vi "大富翁.vi"() -> ()   [LabVIEW 2014] (continued)
                        n3735 = local write "29旅1"(TRUE) -> ()
                      }
                      frame #1 {
                        n3736 = property on="29旅1" class="Bool (strict)"("Visible"=TRUE) -> ()  [unwired: 2 in, 2 out]
                      }
                    }
                  }
                  frame 6 {
                    n3737 = flat-sequence {
                      frame #0 {
                        n3738 = local write "29旅2"(TRUE) -> ()
                      }
                      frame #1 {
                        n3739 = property on="29旅2" class="Bool (strict)"("Visible"=TRUE) -> ()  [unwired: 2 in, 2 out]
                      }
                    }
                  }
                  frame 7 {
                    n3740 = flat-sequence {
                      frame #0 {
                        n3741 = local write "29旅3"(TRUE) -> ()
                      }
                      frame #1 {
                        n3742 = property on="29旅3" class="Bool (strict)"("Visible"=TRUE) -> ()  [unwired: 2 in, 2 out]
                      }
                    }
                  }
                  frame 8 {
                    n3743 = flat-sequence {
                      frame #0 {
                        n3744 = local write "29旅4"(TRUE) -> ()
                      }
                      frame #1 {
                        n3745 = property on="29旅4" class="Bool (strict)"("Visible"=TRUE) -> ()  [unwired: 2 in, 2 out]
                      }
                    }
                  }
                }
                n3746 = case shown="1, Default" w3039 {
                  tunnel: w3043 -> [w3075 w3076 w3077 w3078]
                  frame 1, Default {
                    n3747 = local write "玩家一財產"(w3075) -> ()
                  }
                  frame 2 {
                    n3748 = local write "玩家二財產"(w3076) -> ()
                  }
                  frame 3 {
                    n3749 = local write "玩家三財產"(w3077) -> ()
                  }
                  frame 4 {
                    n3750 = local write "玩家四財產"(w3078) -> ()
                  }
                }
              }
              frame True {
                # "無主地"
                n3751 = call "購買土地.vi"() -> ("確定 2"=w3085:bool)  [unwired: 3 in]
                n3752 = case shown="True" w3085 {
                  tunnel: w3084 -> [_ w3089]
                  frame False {
                    # "不買"
                  }
                  frame True {
                    # "要買"
                    n3753 = local read "換誰?"() -> (w3090:dbl)
                    n3754 = case shown="4" w3090 {
                      tunnel: [w3117 w3118 w3119 w3120] -> w3088
                      frame 1, Default {
                        n3755 = local read "玩家一財產"() -> (w3117:dbl)
                      }
                      frame 2 {
                        n3756 = local read "玩家二財產"() -> (w3118:dbl)
                      }
                      frame 3 {
                        n3757 = local read "玩家三財產"() -> (w3119:dbl)
                      }
                      frame 4 {
                        n3758 = local read "玩家四財產"() -> (w3120:dbl)
                      }
                    }
                    n3759 = call "各種價格.vi"("Numeric"=w3089) -> ("買空地"=w3087:dbl)  [unwired: 4 in, 5 out]
                    n3760 = Greater Or Equal?(x=w3088, y=w3087) -> (x >= y?=w3086:bool)
                    n3761 = case shown="True" w3086 {
                      tunnel: w3089 -> [_ w3091]
                      frame False {
                        # "錢不夠"
                        n3762 = call "錢不夠.vi"() -> ()  [unwired: 4 in]
                      }
                      frame True {
                        # "錢夠"
                        n3763 = local read "換誰?"() -> (w3092:dbl)
                        n3764 = case shown="3" w3092 {
                          selector: w3092 -> [w3096 w3102 w3108 w3114]
                          tunnel: w3091 -> [w3095 w3101 w3107 w3113]
                          frame 1, Default {
                            # "誰買了地"
                            n3765 = call "各種價格.vi"("Numeric"=w3095) -> ("買空地"=w3094:dbl)  [unwired: 4 in, 5 out]
                            n3766 = local read "玩家一財產"() -> (w3098:dbl)
                            n3767 = Subtract(x=w3098, y=w3094) -> (x-y=w3097:dbl)
                            n3768 = local write "玩家一財產"(w3097) -> ()
                            n3769 = call "數字轉顏色.vi"("數字"=w3096) -> ("顏色數字"=w3093:dbl)  [unwired: 2 in]
                            n3770 = local write "29彰化縣"(w3093) -> ()
                            n3771 = local write "彰化縣所有"(w3093) -> ()
                          }
                          frame 2 {
                            # "誰買了地"
                            n3772 = call "各種價格.vi"("Numeric"=w3101) -> ("買空地"=w3100:dbl)  [unwired: 4 in, 5 out]
                            n3773 = local read "玩家二財產"() -> (w3104:dbl)
                            n3774 = Subtract(x=w3104, y=w3100) -> (x-y=w3103:dbl)
                            n3775 = local write "玩家二財產"(w3103) -> ()
                            n3776 = call "數字轉顏色.vi"("數字"=w3102) -> ("顏色數字"=w3099:dbl)  [unwired: 2 in]
                            n3777 = local write "29彰化縣"(w3099) -> ()
                            n3778 = local write "彰化縣所有"(w3099) -> ()
                          }
                          frame 3 {
                            # "誰買了地"
                            n3779 = local read "玩家三財產"() -> (w3109:dbl)
                            n3780 = call "各種價格.vi"("Numeric"=w3107) -> ("買空地"=w3106:dbl)  [unwired: 4 in, 5 out]
                            n3781 = Subtract(x=w3109, y=w3106) -> (x-y=w3110:dbl)
                            n3782 = call "數字轉顏色.vi"("數字"=w3108) -> ("顏色數字"=w3105:dbl)  [unwired: 2 in]
                            n3783 = local write "玩家三財產"(w3110) -> ()
                            n3784 = local write "29彰化縣"(w3105) -> ()
                            n3785 = local write "彰化縣所有"(w3105) -> ()
                          }
                          frame 4 {
                            # "誰買了地"
                            n3786 = call "各種價格.vi"("Numeric"=w3113) -> ("買空地"=w3112:dbl)  [unwired: 4 in, 5 out]
                            n3787 = local read "玩家四財產"() -> (w3116:dbl)
                            n3788 = Subtract(x=w3116, y=w3112) -> (x-y=w3115:dbl)
                            n3789 = local write "玩家四財產"(w3115) -> ()
                            n3790 = call "數字轉顏色.vi"("數字"=w3114) -> ("顏色數字"=w3111:dbl)  [unwired: 2 in]
                            n3791 = local write "29彰化縣"(w3111) -> ()
                            n3792 = local write "彰化縣所有"(w3111) -> ()
                          }
                        }
                      }
                    }
                  }
                }
              }
            }
          }
          frame 30 {
            n3793 = local read "南投縣所有"() -> (w3121:u32)
            n3794 = Equal?(x=w3121, y=u32 16777215) -> (x = y?=w3124:bool)
            n3795 = case shown="False" w3124 {
              tunnel: w3122 -> [w3147 w3185]
              tunnel: [w3137 FALSE] -> w3123
              frame False {
                # "有主地"
                n3796 = local read "換誰?"() -> (w3140:dbl)
                n3797 = local read "南投縣所有"() -> (w3128:u32)
                n3798 = call "數字轉顏色.vi"("數字"=w3140) -> ("顏色數字"=w3151:dbl)  [unwired: 2 in]
                n3799 = case shown="4" w3140 {
                  tunnel: [w3180 w3181 w3182 w3183] -> w3146
                  frame 1, Default {
                    n3800 = local read "玩家一財產"() -> (w3180:dbl)
                  }
                  frame 2 {
                    n3801 = local read "玩家二財產"() -> (w3181:dbl)
                  }
                  frame 3 {
                    n3802 = local read "玩家三財產"() -> (w3182:dbl)
                  }
                  frame 4 {
                    n3803 = local read "玩家四財產"() -> (w3183:dbl)
                  }
                }
                n3804 = Equal?(x=w3128, y=w3151) -> (x = y?=w3150:bool)
                n3805 = local read "30旅4"() -> (w3129:bool)
                n3806 = local read "30旅3"() -> (w3130:bool)
                n3807 = local read "30旅2"() -> (w3131:bool)
                n3808 = local read "30旅1"() -> (w3132:bool)
                n3809 = local read "30房4"() -> (w3133:bool)
                n3810 = local read "30房3"() -> (w3134:bool)
                n3811 = local read "30房2"() -> (w3135:bool)
                n3812 = local read "30房1"() -> (w3136:bool)
                n3813 = local read "南投縣所有"() -> (w3127:u32)
                n3814 = call "房子數量.vi"("房子 1"=w3136, "房子 2"=w3135, "房子 3"=w3134, "房子 4"=w3133, "旅館 1"=w3132, "旅館 2"=w3131, "旅館 3"=w3130, "旅館 4"=w3129) -> ("房子數"=w3149:dbl, "旅館數"=w3148:dbl)  [unwired: 18 in]
                n3815 = call "顏色轉數字.vi"("顏色數字"=w3127) -> ("數字"=w3138:dbl)  [unwired: 2 in]
                n3816 = case shown="1, Default" w3138 {
                  tunnel: [w3156 w3157 w3158 w3159] -> w3142
                  frame 1, Default {
                    n3817 = local read "玩家一財產"() -> (w3156:dbl)
                  }
                  frame 2 {
                    n3818 = local read "玩家二財產"() -> (w3157:dbl)
                  }
                  frame 3 {
                    n3819 = local read "玩家三財產"() -> (w3158:dbl)
                  }
                  frame 4 {
                    n3820 = local read "玩家四財產"() -> (w3159:dbl)
                  }
                }
                n3821 = call "走到地.vi"("房子數量"=w3149, "自己的地?"=w3150, "旅館數量"=w3148, "編號"=w3147, "走到人財產"=w3146) -> ("走到人-?"=w3145:dbl, "蓋第幾棟"=w3143:dbl, "地主+?"=w3141:dbl, "破產?"=w3137:bool)
                n3822 = Subtract(x=w3146, y=w3145) -> (x-y=w3144:dbl)
                n3823 = Add(x=w3141, y=w3142) -> (x+y=w3139:dbl)
                n3824 = case shown="1, Default" w3138 {
                  tunnel: w3139 -> [w3152 w3153 w3154 w3155]
                  frame 1, Default {
                    n3825 = local write "玩家一財產"(w3152) -> ()
                  }
                  frame 2 {
                    n3826 = local write "玩家二財產"(w3153) -> ()
                  }
                  frame 3 {
                    n3827 = local write "玩家三財產"(w3154) -> ()
                  }
                  frame 4 {
                    n3828 = local write "玩家四財產"(w3155) -> ()
                  }
                }
                n3829 = case shown="6" w3143 {
                  frame 0, Default {
                  }
                  frame 1 {
                    n3830 = flat-sequence {
                      frame #0 {
                        n3831 = local write "30房1"(TRUE ("1房1")) -> ()
                      }
                      frame #1 {
                        n3832 = property on="30房1" class="Bool (strict)"("Visible"=TRUE) -> ()  [unwired: 2 in, 2 out]
                      }
                    }
                  }
                  frame 2 {
                    n3833 = flat-sequence {
                      frame #0 {
                        n3834 = local write "30房2"(TRUE ("30房2")) -> ()
                      }
                      frame #1 {
                        n3835 = property on="30房2" class="Bool (strict)"("Visible"=TRUE) -> ()  [unwired: 2 in, 2 out]
                      }
                    }
                  }
                  frame 3 {
                    n3836 = flat-sequence {
                      frame #0 {
                        n3837 = local write "30房3"(TRUE) -> ()
                      }
                      frame #1 {
                        n3838 = property on="30房3" class="Bool (strict)"("Visible"=TRUE) -> ()  [unwired: 2 in, 2 out]
                      }
                    }
                  }
                  frame 4 {
                    n3839 = flat-sequence {
                      frame #0 {
                        n3840 = local write "30房4"(TRUE) -> ()
                      }
                      frame #1 {
                        n3841 = property on="30房4" class="Bool (strict)"("Visible"=TRUE) -> ()  [unwired: 2 in, 2 out]
                      }
                    }
                  }
                  frame 5 {
                    n3842 = flat-sequence {
                      frame #0 {
                        n3843 = local write "30旅1"(TRUE) -> ()
                      }
                      frame #1 {
                        n3844 = property on="30旅1" class="Bool (strict)"("Visible"=TRUE) -> ()  [unwired: 2 in, 2 out]
                      }
                    }
                  }
                  frame 6 {
                    n3845 = flat-sequence {
                      frame #0 {
                        n3846 = local write "30旅2"(TRUE) -> ()
                      }
                      frame #1 {
                        n3847 = property on="30旅2" class="Bool (strict)"("Visible"=TRUE) -> ()  [unwired: 2 in, 2 out]
                      }
                    }
                  }
                  frame 7 {
                    n3848 = flat-sequence {
                      frame #0 {
                        n3849 = local write "30旅3"(TRUE) -> ()
                      }
                      frame #1 {
                        n3850 = property on="30旅3" class="Bool (strict)"("Visible"=TRUE) -> ()  [unwired: 2 in, 2 out]
                      }
                    }
                  }
                  frame 8 {
                    n3851 = flat-sequence {
                      frame #0 {
                        n3852 = local write "30旅4"(TRUE) -> ()
                      }
                      frame #1 {
                        n3853 = property on="30旅4" class="Bool (strict)"("Visible"=TRUE) -> ()  [unwired: 2 in, 2 out]
                      }
                    }
                  }
                }
                n3854 = case shown="1, Default" w3140 {
                  tunnel: w3144 -> [w3176 w3177 w3178 w3179]
                  frame 1, Default {
                    n3855 = local write "玩家一財產"(w3176) -> ()
                  }
                  frame 2 {
                    n3856 = local write "玩家二財產"(w3177) -> ()
                  }
                  frame 3 {
                    n3857 = local write "玩家三財產"(w3178) -> ()
                  }
                  frame 4 {
                    n3858 = local write "玩家四財產"(w3179) -> ()
                  }
                }
              }
              frame True {
                # "無主地"
                n3859 = call "購買土地.vi"() -> ("確定 2"=w3186:bool)  [unwired: 3 in]
                n3860 = case shown="True" w3186 {
                  tunnel: w3185 -> [_ w3190]
                  frame False {
                    # "不買"
                  }
                  frame True {
                    # "要買"
                    n3861 = local read "換誰?"() -> (w3191:dbl)
                    n3862 = case shown="4" w3191 {
                      tunnel: [w3218 w3219 w3220 w3221] -> w3189
                      frame 1, Default {
                        n3863 = local read "玩家一財產"() -> (w3218:dbl)
                      }
                      frame 2 {
                        n3864 = local read "玩家二財產"() -> (w3219:dbl)
                      }
                      frame 3 {
                        n3865 = local read "玩家三財產"() -> (w3220:dbl)
                      }
                      frame 4 {
                        n3866 = local read "玩家四財產"() -> (w3221:dbl)
                      }
                    }
                    n3867 = call "各種價格.vi"("Numeric"=w3190) -> ("買空地"=w3188:dbl)  [unwired: 4 in, 5 out]
                    n3868 = Greater Or Equal?(x=w3189, y=w3188) -> (x >= y?=w3187:bool)
                    n3869 = case shown="True" w3187 {
                      tunnel: w3190 -> [_ w3192]
                      frame False {
                        # "錢不夠"
                        n3870 = call "錢不夠.vi"() -> ()  [unwired: 4 in]
                      }
                      frame True {
                        # "錢夠"
                        n3871 = local read "換誰?"() -> (w3193:dbl)
                        n3872 = case shown="4" w3193 {
                          selector: w3193 -> [w3197 w3203 w3209 w3215]
                          tunnel: w3192 -> [w3196 w3202 w3208 w3214]
                          frame 1, Default {
                            # "誰買了地"
                            n3873 = call "各種價格.vi"("Numeric"=w3196) -> ("買空地"=w3195:dbl)  [unwired: 4 in, 5 out]
                            n3874 = local read "玩家一財產"() -> (w3199:dbl)
                            n3875 = Subtract(x=w3199, y=w3195) -> (x-y=w3198:dbl)
                            n3876 = local write "玩家一財產"(w3198) -> ()
                            n3877 = call "數字轉顏色.vi"("數字"=w3197) -> ("顏色數字"=w3194:dbl)  [unwired: 2 in]
                            n3878 = local write "30南投縣"(w3194) -> ()
                            n3879 = local write "南投縣所有"(w3194) -> ()
                          }
                          frame 2 {
                            # "誰買了地"
                            n3880 = call "各種價格.vi"("Numeric"=w3202) -> ("買空地"=w3201:dbl)  [unwired: 4 in, 5 out]
                            n3881 = local read "玩家二財產"() -> (w3205:dbl)
                            n3882 = Subtract(x=w3205, y=w3201) -> (x-y=w3204:dbl)
                            n3883 = local write "玩家二財產"(w3204) -> ()
                            n3884 = call "數字轉顏色.vi"("數字"=w3203) -> ("顏色數字"=w3200:dbl)  [unwired: 2 in]
                            n3885 = local write "30南投縣"(w3200) -> ()
                            n3886 = local write "南投縣所有"(w3200) -> ()
                          }
                          frame 3 {
                            # "誰買了地"
                            n3887 = local read "玩家三財產"() -> (w3210:dbl)
                            n3888 = call "各種價格.vi"("Numeric"=w3208) -> ("買空地"=w3207:dbl)  [unwired: 4 in, 5 out]
                            n3889 = Subtract(x=w3210, y=w3207) -> (x-y=w3211:dbl)
                            n3890 = call "數字轉顏色.vi"("數字"=w3209) -> ("顏色數字"=w3206:dbl)  [unwired: 2 in]
                            n3891 = local write "玩家三財產"(w3211) -> ()
                            n3892 = local write "30南投縣"(w3206) -> ()
                            n3893 = local write "南投縣所有"(w3206) -> ()
                          }
                          frame 4 {
                            # "誰買了地"
                            n3894 = call "各種價格.vi"("Numeric"=w3214) -> ("買空地"=w3213:dbl)  [unwired: 4 in, 5 out]
                            n3895 = local read "玩家四財產"() -> (w3217:dbl)
                            n3896 = Subtract(x=w3217, y=w3213) -> (x-y=w3216:dbl)
                            n3897 = local write "玩家四財產"(w3216) -> ()
                            n3898 = call "數字轉顏色.vi"("數字"=w3215) -> ("顏色數字"=w3212:dbl)  [unwired: 2 in]
                            n3899 = local write "30南投縣"(w3212) -> ()
                            n3900 = local write "南投縣所有"(w3212) -> ()
                          }
                        }
                      }
                    }
                  }
                }
              }
            }
          }
          frame 31 {
            n3901 = local read "台中市所有"() -> (w3222:u32)
            n3902 = Equal?(x=w3222, y=u32 16777215) -> (x = y?=w3225:bool)
            n3903 = case shown="True" w3225 {
              tunnel: w3224 -> [w3248 w3286]
              tunnel: [w3238 FALSE] -> w3223
              frame False {
                # "有主地"
                n3904 = local read "換誰?"() -> (w3241:dbl)
                n3905 = local read "台中市所有"() -> (w3229:u32)
                n3906 = call "數字轉顏色.vi"("數字"=w3241) -> ("顏色數字"=w3252:dbl)  [unwired: 2 in]
                n3907 = case shown="4" w3241 {
                  tunnel: [w3281 w3282 w3283 w3284] -> w3247
                  frame 1, Default {
                    n3908 = local read "玩家一財產"() -> (w3281:dbl)
                  }
                  frame 2 {
                    n3909 = local read "玩家二財產"() -> (w3282:dbl)
                  }
                  frame 3 {
                    n3910 = local read "玩家三財產"() -> (w3283:dbl)
                  }
                  frame 4 {
                    n3911 = local read "玩家四財產"() -> (w3284:dbl)
                  }
                }
                n3912 = Equal?(x=w3229, y=w3252) -> (x = y?=w3251:bool)
                n3913 = local read "31旅4"() -> (w3230:bool)
                n3914 = local read "31旅3"() -> (w3231:bool)
                n3915 = local read "31旅2"() -> (w3232:bool)
                n3916 = local read "31旅1"() -> (w3233:bool)
                n3917 = local read "31房4"() -> (w3234:bool)
                n3918 = local read "31房3"() -> (w3235:bool)
                n3919 = local read "31房2"() -> (w3236:bool)
                n3920 = local read "31房1"() -> (w3237:bool)
                n3921 = local read "台中市所有"() -> (w3228:u32)
                n3922 = call "房子數量.vi"("房子 1"=w3237, "房子 2"=w3236, "房子 3"=w3235, "房子 4"=w3234, "旅館 1"=w3233, "旅館 2"=w3232, "旅館 3"=w3231, "旅館 4"=w3230) -> ("房子數"=w3250:dbl, "旅館數"=w3249:dbl)  [unwired: 18 in]
                n3923 = call "顏色轉數字.vi"("顏色數字"=w3228) -> ("數字"=w3239:dbl)  [unwired: 2 in]
                n3924 = case shown="1, Default" w3239 {
                  tunnel: [w3257 w3258 w3259 w3260] -> w3243
                  frame 1, Default {
                    n3925 = local read "玩家一財產"() -> (w3257:dbl)
                  }
                  frame 2 {
                    n3926 = local read "玩家二財產"() -> (w3258:dbl)
                  }
                  frame 3 {
                    n3927 = local read "玩家三財產"() -> (w3259:dbl)
                  }
                  frame 4 {
                    n3928 = local read "玩家四財產"() -> (w3260:dbl)
                  }
                }
                n3929 = call "走到地.vi"("房子數量"=w3250, "自己的地?"=w3251, "旅館數量"=w3249, "編號"=w3248, "走到人財產"=w3247) -> ("走到人-?"=w3246:dbl, "蓋第幾棟"=w3244:dbl, "地主+?"=w3242:dbl, "破產?"=w3238:bool)
                n3930 = Subtract(x=w3247, y=w3246) -> (x-y=w3245:dbl)
                n3931 = Add(x=w3242, y=w3243) -> (x+y=w3240:dbl)
                n3932 = case shown="1, Default" w3239 {
                  tunnel: w3240 -> [w3253 w3254 w3255 w3256]
                  frame 1, Default {
                    n3933 = local write "玩家一財產"(w3253) -> ()
                  }
                  frame 2 {
                    n3934 = local write "玩家二財產"(w3254) -> ()
                  }
                  frame 3 {
                    n3935 = local write "玩家三財產"(w3255) -> ()
                  }
                  frame 4 {
                    n3936 = local write "玩家四財產"(w3256) -> ()
                  }
                }
                n3937 = case shown="1" w3244 {
                  frame 0, Default {
                  }
                  frame 1 {
                    n3938 = flat-sequence {
                      frame #0 {
                        n3939 = local write "31房1"(TRUE ("1房1")) -> ()
                      }
                      frame #1 {
                        n3940 = property on="31房1" class="Bool (strict)"("Visible"=TRUE) -> ()  [unwired: 2 in, 2 out]
                      }
                    }
                  }
                  frame 2 {
                    n3941 = flat-sequence {
                      frame #0 {
                        n3942 = local write "31房2"(TRUE ("1房2")) -> ()
                      }
                      frame #1 {
                        n3943 = property on="31房2" class="Bool (strict)"("Visible"=TRUE ("1房2")) -> ()  [unwired: 2 in, 2 out]
                      }
                    }
                  }
                  frame 3 {
                    n3944 = flat-sequence {
                      frame #0 {
                        n3945 = local write "31房3"(TRUE) -> ()
                      }
                      frame #1 {
                        n3946 = property on="31房3" class="Bool (strict)"("Visible"=TRUE) -> ()  [unwired: 2 in, 2 out]
                      }
                    }
                  }
                  frame 4 {
                    n3947 = flat-sequence {
                      frame #0 {
                        n3948 = local write "31房4"(TRUE) -> ()
                      }
                      frame #1 {
                        n3949 = property on="31房4" class="Bool (strict)"("Visible"=TRUE) -> ()  [unwired: 2 in, 2 out]
                      }
                    }
                  }
                  frame 5 {
                    n3950 = flat-sequence {
                      frame #0 {
                        n3951 = local write "31旅1"(TRUE) -> ()
                      }
                      frame #1 {
                        n3952 = property on="31旅1" class="Bool (strict)"("Visible"=TRUE) -> ()  [unwired: 2 in, 2 out]
                      }
                    }
                  }
                  frame 6 {
                    n3953 = flat-sequence {
                      frame #0 {
                        n3954 = local write "31旅2"(TRUE) -> ()
                      }
                      frame #1 {
                        n3955 = property on="31旅2" class="Bool (strict)"("Visible"=TRUE) -> ()  [unwired: 2 in, 2 out]
                      }
                    }
                  }
                  frame 7 {
                    n3956 = flat-sequence {
                      frame #0 {
                        n3957 = local write "31旅3"(TRUE) -> ()
                      }
                      frame #1 {
                        n3958 = property on="31旅3" class="Bool (strict)"("Visible"=TRUE) -> ()  [unwired: 2 in, 2 out]
                      }
                    }
                  }
                  frame 8 {
                    n3959 = flat-sequence {
                      frame #0 {
                        n3960 = local write "31旅4"(TRUE) -> ()
                      }
                      frame #1 {
                        n3961 = property on="31旅4" class="Bool (strict)"("Visible"=TRUE) -> ()  [unwired: 2 in, 2 out]
                      }
                    }
                  }
                }
                n3962 = case shown="1, Default" w3241 {
                  tunnel: w3245 -> [w3277 w3278 w3279 w3280]
                  frame 1, Default {
                    n3963 = local write "玩家一財產"(w3277) -> ()
                  }
                  frame 2 {
                    n3964 = local write "玩家二財產"(w3278) -> ()
                  }
                  frame 3 {
                    n3965 = local write "玩家三財產"(w3279) -> ()
                  }
                  frame 4 {
                    n3966 = local write "玩家四財產"(w3280) -> ()
                  }
                }
              }
              frame True {
                # "無主地"
                n3967 = call "購買土地.vi"() -> ("確定 2"=w3287:bool)  [unwired: 3 in]
                n3968 = case shown="True" w3287 {
                  tunnel: w3286 -> [_ w3291]
                  frame False {
                    # "不買"
                  }
                  frame True {
                    # "要買"
                    n3969 = local read "換誰?"() -> (w3292:dbl)
                    n3970 = case shown="4" w3292 {
                      tunnel: [w3319 w3320 w3321 w3322] -> w3290
                      frame 1, Default {
                        n3971 = local read "玩家一財產"() -> (w3319:dbl)
                      }
                      frame 2 {
                        n3972 = local read "玩家二財產"() -> (w3320:dbl)
                      }
                      frame 3 {
                        n3973 = local read "玩家三財產"() -> (w3321:dbl)
                      }
                      frame 4 {
                        n3974 = local read "玩家四財產"() -> (w3322:dbl)
                      }
                    }
                    n3975 = call "各種價格.vi"("Numeric"=w3291) -> ("買空地"=w3289:dbl)  [unwired: 4 in, 5 out]
                    n3976 = Greater Or Equal?(x=w3290, y=w3289) -> (x >= y?=w3288:bool)
                    n3977 = case shown="True" w3288 {
                      tunnel: w3291 -> [_ w3293]
                      frame False {
                        # "錢不夠"
                        n3978 = call "錢不夠.vi"() -> ()  [unwired: 4 in]
                      }
                      frame True {
                        # "錢夠"
                        n3979 = local read "換誰?"() -> (w3294:dbl)
                        n3980 = case shown="1, Default" w3294 {
                          selector: w3294 -> [w3298 w3304 w3310 w3316]
                          tunnel: w3293 -> [w3297 w3303 w3309 w3315]
                          frame 1, Default {
                            # "誰買了地"
                            n3981 = call "各種價格.vi"("Numeric"=w3297) -> ("買空地"=w3296:dbl)  [unwired: 4 in, 5 out]
                            n3982 = local read "玩家一財產"() -> (w3300:dbl)
                            n3983 = Subtract(x=w3300, y=w3296) -> (x-y=w3299:dbl)
                            n3984 = local write "玩家一財產"(w3299) -> ()
                            n3985 = call "數字轉顏色.vi"("數字"=w3298) -> ("顏色數字"=w3295:dbl)  [unwired: 2 in]
                            n3986 = local write "31台中市"(w3295) -> ()
                            n3987 = local write "台中市所有"(w3295) -> ()
                          }
                          frame 2 {
                            # "誰買了地"
                            n3988 = call "各種價格.vi"("Numeric"=w3303) -> ("買空地"=w3302:dbl)  [unwired: 4 in, 5 out]
                            n3989 = local read "玩家二財產"() -> (w3306:dbl)
                            n3990 = Subtract(x=w3306, y=w3302) -> (x-y=w3305:dbl)
                            n3991 = local write "玩家二財產"(w3305) -> ()
                            n3992 = call "數字轉顏色.vi"("數字"=w3304) -> ("顏色數字"=w3301:dbl)  [unwired: 2 in]
                            n3993 = local write "31台中市"(w3301) -> ()
                            n3994 = local write "台中市所有"(w3301) -> ()
                          }
                          frame 3 {
                            # "誰買了地"
                            n3995 = local read "玩家三財產"() -> (w3311:dbl)
                            n3996 = call "各種價格.vi"("Numeric"=w3309) -> ("買空地"=w3308:dbl)  [unwired: 4 in, 5 out]
                            n3997 = Subtract(x=w3311, y=w3308) -> (x-y=w3312:dbl)
                            n3998 = call "數字轉顏色.vi"("數字"=w3310) -> ("顏色數字"=w3307:dbl)  [unwired: 2 in]
                            n3999 = local write "玩家三財產"(w3312) -> ()
                            n4000 = local write "31台中市"(w3307) -> ()
                            n4001 = local write "台中市所有"(w3307) -> ()
                          }
                          frame 4 {
                            # "誰買了地"
                            n4002 = call "各種價格.vi"("Numeric"=w3315) -> ("買空地"=w3314:dbl)  [unwired: 4 in, 5 out]
                            n4003 = local read "玩家四財產"() -> (w3318:dbl)
                            n4004 = Subtract(x=w3318, y=w3314) -> (x-y=w3317:dbl)
                            n4005 = local write "玩家四財產"(w3317) -> ()
                            n4006 = call "數字轉顏色.vi"("數字"=w3316) -> ("顏色數字"=w3313:dbl)  [unwired: 2 in]
                            n4007 = local write "31台中市"(w3313) -> ()
                            n4008 = local write "台中市所有"(w3313) -> ()
                          }
                        }
                      }
                    }
                  }
                }
              }
            }
          }
          frame 32 {
            n4009 = local read "換誰?"() -> (w3323:dbl)
            n4010 = case shown="4" w3323 {
              frame 0, Default {
              }
              frame 1 {
                n4011 = local write "剩幾天 1"(2.0 ("剩幾天 1")) -> ()
                n4012 = local write "位置 1"(13.0 ("位置 1")) -> ()
                n4013 = property on="入獄 1" class="Bool (strict)"("Visible"=TRUE) -> ()  [unwired: 2 in, 2 out]
                n4014 = property on="P1 棋子" class="Bool (strict)"("Left"=1503 ("Position:Left"), "Top"=112 ("Position:Top")) -> ()  [unwired: 2 in, 2 out]
              }
              frame 2 {
                n4015 = local write "剩幾天 2"(2.0 ("剩幾天 2")) -> ()
                n4016 = local write "位置 2"(13.0 ("位置 2")) -> ()
                n4017 = property on="入獄 2" class="Bool (strict)"("Visible"=TRUE) -> ()  [unwired: 2 in, 2 out]
                n4018 = property on="P2 棋子" class="Bool (strict)"("Left"=1540 ("Position:Left"), "Top"=112 ("Position:Top")) -> ()  [unwired: 2 in, 2 out]
              }
              frame 3 {
                n4019 = local write "剩幾天 3"(2.0 ("剩幾天 3")) -> ()
                n4020 = local write "位置 3"(13.0 ("位置 3")) -> ()
                n4021 = property on="入獄 3" class="Bool (strict)"("Visible"=TRUE) -> ()  [unwired: 2 in, 2 out]
                n4022 = property on="P3 棋子" class="Bool (strict)"("Left"=1503 ("Position:Left"), "Top"=144 ("Position:Top")) -> ()  [unwired: 2 in, 2 out]
              }
              frame 4 {
                n4023 = local write "剩幾天 4"(2.0 ("剩幾天 4")) -> ()
                n4024 = property on="入獄 4" class="Bool (strict)"("Visible"=TRUE) -> ()  [unwired: 2 in, 2 out]
                n4025 = local write "位置 4"(13.0 ("位置 4")) -> ()
                n4026 = property on="P4 棋子" class="Bool (strict)"("Left"=1540 ("Position:Left"), "Top"=144 ("Position:Top")) -> ()  [unwired: 2 in, 2 out]
              }
            }
            n4027 = call "32入獄.vi"() -> ()  [unwired: 4 in]
          }
          frame 33 {
            n4028 = local read "苗栗縣所有"() -> (w3346:u32)
            n4029 = Equal?(x=w3346, y=u32 16777215) -> (x = y?=w3349:bool)
            n4030 = case shown="True" w3349 {
              tunnel: w3348 -> [w3372 w3410]
              tunnel: [w3362 FALSE] -> w3347
              frame False {
                # "有主地"
                n4031 = local read "換誰?"() -> (w3365:dbl)
                n4032 = local read "苗栗縣所有"() -> (w3353:u32)
                n4033 = call "數字轉顏色.vi"("數字"=w3365) -> ("顏色數字"=w3376:dbl)  [unwired: 2 in]
                n4034 = case shown="4" w3365 {
                  tunnel: [w3405 w3406 w3407 w3408] -> w3371
                  frame 1, Default {
                    n4035 = local read "玩家一財產"() -> (w3405:dbl)
                  }
                  frame 2 {
                    n4036 = local read "玩家二財產"() -> (w3406:dbl)
                  }
                  frame 3 {
                    n4037 = local read "玩家三財產"() -> (w3407:dbl)
                  }
                  frame 4 {
                    n4038 = local read "玩家四財產"() -> (w3408:dbl)
                  }
                }
                n4039 = Equal?(x=w3353, y=w3376) -> (x = y?=w3375:bool)
                n4040 = local read "33旅4"() -> (w3354:bool)
                n4041 = local read "33旅3"() -> (w3355:bool)
                n4042 = local read "33旅2"() -> (w3356:bool)
                n4043 = local read "33旅1"() -> (w3357:bool)
                n4044 = local read "33房4"() -> (w3358:bool)
                n4045 = local read "33房3"() -> (w3359:bool)
                n4046 = local read "33房2"() -> (w3360:bool)
                n4047 = local read "33房1"() -> (w3361:bool)
                n4048 = local read "苗栗縣所有"() -> (w3352:u32)
                n4049 = call "房子數量.vi"("房子 1"=w3361, "房子 2"=w3360, "房子 3"=w3359, "房子 4"=w3358, "旅館 1"=w3357, "旅館 2"=w3356, "旅館 3"=w3355, "旅館 4"=w3354) -> ("房子數"=w3374:dbl, "旅館數"=w3373:dbl)  [unwired: 18 in]
                n4050 = call "顏色轉數字.vi"("顏色數字"=w3352) -> ("數字"=w3363:dbl)  [unwired: 2 in]
                n4051 = case shown="1, Default" w3363 {
                  tunnel: [w3381 w3382 w3383 w3384] -> w3367
                  frame 1, Default {
                    n4052 = local read "玩家一財產"() -> (w3381:dbl)
                  }
                  frame 2 {
                    n4053 = local read "玩家二財產"() -> (w3382:dbl)
                  }
                  frame 3 {
                    n4054 = local read "玩家三財產"() -> (w3383:dbl)
                  }
                  frame 4 {
                    n4055 = local read "玩家四財產"() -> (w3384:dbl)
                  }
                }
                n4056 = call "走到地.vi"("房子數量"=w3374, "自己的地?"=w3375, "旅館數量"=w3373, "編號"=w3372, "走到人財產"=w3371) -> ("走到人-?"=w3370:dbl, "蓋第幾棟"=w3368:dbl, "地主+?"=w3366:dbl, "破產?"=w3362:bool)
                n4057 = Subtract(x=w3371, y=w3370) -> (x-y=w3369:dbl)
                n4058 = Add(x=w3366, y=w3367) -> (x+y=w3364:dbl)
                n4059 = case shown="1, Default" w3363 {
                  tunnel: w3364 -> [w3377 w3378 w3379 w3380]
                  frame 1, Default {
                    n4060 = local write "玩家一財產"(w3377) -> ()
                  }
                  frame 2 {
                    n4061 = local write "玩家二財產"(w3378) -> ()
                  }
                  frame 3 {
                    n4062 = local write "玩家三財產"(w3379) -> ()
                  }
                  frame 4 {
                    n4063 = local write "玩家四財產"(w3380) -> ()
                  }
                }
                n4064 = case shown="5" w3368 {
                  frame 0, Default {
                  }
                  frame 1 {
                    n4065 = flat-sequence {
                      frame #0 {
                        n4066 = local write "33房1"(TRUE ("1房1")) -> ()
                      }
                      frame #1 {
                        n4067 = property on="33房1" class="Bool (strict)"("Visible"=TRUE) -> ()  [unwired: 2 in, 2 out]
                      }
                    }
                  }
                  frame 2 {
                    n4068 = flat-sequence {
                      frame #0 {
                        n4069 = local write "33房2"(TRUE ("1房2")) -> ()
                      }
                      frame #1 {
                        n4070 = property on="33房2" class="Bool (strict)"("Visible"=TRUE ("1房2")) -> ()  [unwired: 2 in, 2 out]
                      }
                    }
                  }
                  frame 3 {
                    n4071 = flat-sequence {
                      frame #0 {
                        n4072 = local write "33房3"(TRUE) -> ()
                      }
                      frame #1 {
                        n4073 = property on="33房3" class="Bool (strict)"("Visible"=TRUE) -> ()  [unwired: 2 in, 2 out]
                      }
                    }
                  }
                  frame 4 {
                    n4074 = flat-sequence {
                      frame #0 {
                        n4075 = local write "33房4"(TRUE) -> ()
                      }
                      frame #1 {
                        n4076 = property on="33房4" class="Bool (strict)"("Visible"=TRUE) -> ()  [unwired: 2 in, 2 out]
                      }
                    }
                  }
                  frame 5 {
                    n4077 = flat-sequence {
                      frame #0 {
                        n4078 = local write "33旅1"(TRUE) -> ()
                      }
                      frame #1 {
                        n4079 = property on="33旅1" class="Bool (strict)"("Visible"=TRUE) -> ()  [unwired: 2 in, 2 out]
                      }
                    }
                  }
                  frame 6 {
                    n4080 = flat-sequence {
                      frame #0 {
                        n4081 = local write "33旅2"(TRUE) -> ()
                      }
                      frame #1 {
                        n4082 = property on="33旅2" class="Bool (strict)"("Visible"=TRUE) -> ()  [unwired: 2 in, 2 out]
                      }
                    }
                  }
                  frame 7 {
                    n4083 = flat-sequence {
                      frame #0 {
                        n4084 = local write "33旅3"(TRUE) -> ()
                      }
                      frame #1 {
                        n4085 = property on="33旅3" class="Bool (strict)"("Visible"=TRUE) -> ()  [unwired: 2 in, 2 out]
                      }
                    }
                  }
                  frame 8 {
                    n4086 = flat-sequence {
                      frame #0 {
                        n4087 = local write "33旅4"(TRUE) -> ()
                      }
                      frame #1 {
                        n4088 = property on="33旅4" class="Bool (strict)"("Visible"=TRUE) -> ()  [unwired: 2 in, 2 out]
                      }
                    }
                  }
                }
                n4089 = case shown="1, Default" w3365 {
                  tunnel: w3369 -> [w3401 w3402 w3403 w3404]
                  frame 1, Default {
                    n4090 = local write "玩家一財產"(w3401) -> ()
                  }
                  frame 2 {
                    n4091 = local write "玩家二財產"(w3402) -> ()
                  }
                  frame 3 {
                    n4092 = local write "玩家三財產"(w3403) -> ()
                  }
                  frame 4 {
                    n4093 = local write "玩家四財產"(w3404) -> ()
                  }
                }
              }
              frame True {
                # "無主地"
                n4094 = call "購買土地.vi"() -> ("確定 2"=w3411:bool)  [unwired: 3 in]
                n4095 = case shown="True" w3411 {
                  tunnel: w3410 -> [_ w3415]
                  frame False {
                    # "不買"
                  }
                  frame True {
                    # "要買"
                    n4096 = local read "換誰?"() -> (w3416:dbl)
                    n4097 = case shown="4" w3416 {
                      tunnel: [w3443 w3444 w3445 w3446] -> w3414
                      frame 1, Default {
                        n4098 = local read "玩家一財產"() -> (w3443:dbl)
                      }
                      frame 2 {
                        n4099 = local read "玩家二財產"() -> (w3444:dbl)
                      }
                      frame 3 {
                        n4100 = local read "玩家三財產"() -> (w3445:dbl)
                      }
                      frame 4 {
                        n4101 = local read "玩家四財產"() -> (w3446:dbl)
                      }
                    }
                    n4102 = call "各種價格.vi"("Numeric"=w3415) -> ("買空地"=w3413:dbl)  [unwired: 4 in, 5 out]
                    n4103 = Greater Or Equal?(x=w3414, y=w3413) -> (x >= y?=w3412:bool)
                    n4104 = case shown="True" w3412 {
                      tunnel: w3415 -> [_ w3417]
                      frame False {
                        # "錢不夠"
                        n4105 = call "錢不夠.vi"() -> ()  [unwired: 4 in]
                      }
                      frame True {
                        # "錢夠"
                        n4106 = local read "換誰?"() -> (w3418:dbl)
                        n4107 = case shown="3" w3418 {
                          selector: w3418 -> [w3422 w3428 w3434 w3440]
                          tunnel: w3417 -> [w3421 w3427 w3433 w3439]
                          frame 1, Default {
                            # "誰買了地"
                            n4108 = call "各種價格.vi"("Numeric"=w3421) -> ("買空地"=w3420:dbl)  [unwired: 4 in, 5 out]
                            n4109 = local read "玩家一財產"() -> (w3424:dbl)
                            n4110 = Subtract(x=w3424, y=w3420) -> (x-y=w3423:dbl)
                            n4111 = local write "玩家一財產"(w3423) -> ()
                            n4112 = call "數字轉顏色.vi"("數字"=w3422) -> ("顏色數字"=w3419:dbl)  [unwired: 2 in]
                            n4113 = local write "33苗栗縣"(w3419) -> ()
                            n4114 = local write "苗栗縣所有"(w3419) -> ()
                          }
                          frame 2 {
                            # "誰買了地"
                            n4115 = call "各種價格.vi"("Numeric"=w3427) -> ("買空地"=w3426:dbl)  [unwired: 4 in, 5 out]
                            n4116 = local read "玩家二財產"() -> (w3430:dbl)
                            n4117 = Subtract(x=w3430, y=w3426) -> (x-y=w3429:dbl)
                            n4118 = local write "玩家二財產"(w3429) -> ()
                            n4119 = call "數字轉顏色.vi"("數字"=w3428) -> ("顏色數字"=w3425:dbl)  [unwired: 2 in]
                            n4120 = local write "33苗栗縣"(w3425) -> ()
                            n4121 = local write "苗栗縣所有"(w3425) -> ()
                          }
                          frame 3 {
                            # "誰買了地"
                            n4122 = local read "玩家三財產"() -> (w3435:dbl)
                            n4123 = call "各種價格.vi"("Numeric"=w3433) -> ("買空地"=w3432:dbl)  [unwired: 4 in, 5 out]
                            n4124 = Subtract(x=w3435, y=w3432) -> (x-y=w3436:dbl)
                            n4125 = call "數字轉顏色.vi"("數字"=w3434) -> ("顏色數字"=w3431:dbl)  [unwired: 2 in]
                            n4126 = local write "玩家三財產"(w3436) -> ()
                            n4127 = local write "33苗栗縣"(w3431) -> ()
                            n4128 = local write "苗栗縣所有"(w3431) -> ()
                          }
                          frame 4 {
                            # "誰買了地"
                            n4129 = call "各種價格.vi"("Numeric"=w3439) -> ("買空地"=w3438:dbl)  [unwired: 4 in, 5 out]
                            n4130 = local read "玩家四財產"() -> (w3442:dbl)
                            n4131 = Subtract(x=w3442, y=w3438) -> (x-y=w3441:dbl)
                            n4132 = local write "玩家四財產"(w3441) -> ()
                            n4133 = call "數字轉顏色.vi"("數字"=w3440) -> ("顏色數字"=w3437:dbl)  [unwired: 2 in]
                            n4134 = local write "33苗栗縣"(w3437) -> ()
                            n4135 = local write "苗栗縣所有"(w3437) -> ()
                          }
                        }
                      }
                    }
                  }
                }
              }
            }
          }
          frame 34 {
            n4136 = local read "新竹縣所有"() -> (w3447:u32)
            n4137 = Equal?(x=w3447, y=u32 16777215) -> (x = y?=w3450:bool)
            n4138 = case shown="False" w3450 {
              tunnel: w3449 -> [w3473 w3511]
              tunnel: [w3463 FALSE] -> w3448
              frame False {
                # "有主地"
                n4139 = local read "換誰?"() -> (w3466:dbl)
                n4140 = local read "新竹縣所有"() -> (w3454:u32)
                n4141 = call "數字轉顏色.vi"("數字"=w3466) -> ("顏色數字"=w3477:dbl)  [unwired: 2 in]
                n4142 = case shown="1, Default" w3466 {
                  tunnel: [w3506 w3507 w3508 w3509] -> w3472
                  frame 1, Default {
                    n4143 = local read "玩家一財產"() -> (w3506:dbl)
                  }
                  frame 2 {
                    n4144 = local read "玩家二財產"() -> (w3507:dbl)
                  }
                  frame 3 {
                    n4145 = local read "玩家三財產"() -> (w3508:dbl)
                  }
                  frame 4 {
                    n4146 = local read "玩家四財產"() -> (w3509:dbl)
                  }
                }
                n4147 = Equal?(x=w3454, y=w3477) -> (x = y?=w3476:bool)
                n4148 = local read "34旅4"() -> (w3455:bool)
                n4149 = local read "34旅3"() -> (w3456:bool)
                n4150 = local read "34旅2"() -> (w3457:bool)
                n4151 = local read "34旅1"() -> (w3458:bool)
                n4152 = local read "34房4"() -> (w3459:bool)
                n4153 = local read "34房3"() -> (w3460:bool)
                n4154 = local read "34房2"() -> (w3461:bool)
                n4155 = local read "34房1"() -> (w3462:bool)
                n4156 = local read "新竹縣所有"() -> (w3453:u32)
                n4157 = call "房子數量.vi"("房子 1"=w3462, "房子 2"=w3461, "房子 3"=w3460, "房子 4"=w3459, "旅館 1"=w3458, "旅館 2"=w3457, "旅館 3"=w3456, "旅館 4"=w3455) -> ("房子數"=w3475:dbl, "旅館數"=w3474:dbl)  [unwired: 18 in]
                n4158 = call "顏色轉數字.vi"("顏色數字"=w3453) -> ("數字"=w3464:dbl)  [unwired: 2 in]
                n4159 = case shown="1, Default" w3464 {
                  tunnel: [w3482 w3483 w3484 w3485] -> w3468
                  frame 1, Default {
                    n4160 = local read "玩家一財產"() -> (w3482:dbl)
                  }
                  frame 2 {
                    n4161 = local read "玩家二財產"() -> (w3483:dbl)
                  }
                  frame 3 {
                    n4162 = local read "玩家三財產"() -> (w3484:dbl)
                  }
                  frame 4 {
                    n4163 = local read "玩家四財產"() -> (w3485:dbl)
                  }
                }
                n4164 = call "走到地.vi"("房子數量"=w3475, "自己的地?"=w3476, "旅館數量"=w3474, "編號"=w3473, "走到人財產"=w3472) -> ("走到人-?"=w3471:dbl, "蓋第幾棟"=w3469:dbl, "地主+?"=w3467:dbl, "破產?"=w3463:bool)
                n4165 = Subtract(x=w3472, y=w3471) -> (x-y=w3470:dbl)
                n4166 = Add(x=w3467, y=w3468) -> (x+y=w3465:dbl)
                n4167 = case shown="1, Default" w3466 {
                  tunnel: w3470 -> [w3502 w3503 w3504 w3505]
                  frame 1, Default {
                    n4168 = local write "玩家一財產"(w3502) -> ()
                  }
                  frame 2 {
                    n4169 = local write "玩家二財產"(w3503) -> ()
                  }
                  frame 3 {
                    n4170 = local write "玩家三財產"(w3504) -> ()
                  }
                  frame 4 {
                    n4171 = local write "玩家四財產"(w3505) -> ()
                  }
                }
                n4172 = case shown="1" w3469 {
                  frame 0, Default {
                  }
                  frame 1 {
                    n4173 = flat-sequence {
                      frame #0 {
                        n4174 = local write "34房1"(TRUE ("1房1")) -> ()
                      }
                      frame #1 {
                        n4175 = property on="34房1" class="Bool (strict)"("Visible"=TRUE) -> ()  [unwired: 2 in, 2 out]
                      }
                    }
                  }
                  frame 2 {
                    n4176 = flat-sequence {
                      frame #0 {
                        n4177 = local write "34房2"(TRUE ("1房2")) -> ()
                      }
                      frame #1 {
                        n4178 = property on="34房2" class="Bool (strict)"("Visible"=TRUE ("1房2")) -> ()  [unwired: 2 in, 2 out]
                      }
                    }
                  }
                  frame 3 {
                    n4179 = flat-sequence {
                      frame #0 {
                        n4180 = local write "34房3"(TRUE) -> ()
                      }
                      frame #1 {
                        n4181 = property on="34房3" class="Bool (strict)"("Visible"=TRUE) -> ()  [unwired: 2 in, 2 out]
                      }
                    }
                  }
                  frame 4 {
                    n4182 = flat-sequence {
                      frame #0 {
                        n4183 = local write "34房4"(TRUE) -> ()
                      }
                      frame #1 {
                        n4184 = property on="34房4" class="Bool (strict)"("Visible"=TRUE) -> ()  [unwired: 2 in, 2 out]
                      }
                    }
                  }
                  frame 5 {
                    n4185 = flat-sequence {
                      frame #0 {
                        n4186 = local write "34旅1"(TRUE) -> ()
                      }
                      frame #1 {
                        n4187 = property on="34旅1" class="Bool (strict)"("Visible"=TRUE) -> ()  [unwired: 2 in, 2 out]
                      }
                    }
                  }
                  frame 6 {
                    n4188 = flat-sequence {
                      frame #0 {
                        n4189 = local write "34旅2"(TRUE) -> ()
                      }
                      frame #1 {
                        n4190 = property on="34旅2" class="Bool (strict)"("Visible"=TRUE) -> ()  [unwired: 2 in, 2 out]
                      }
                    }
                  }
                  frame 7 {
                    n4191 = flat-sequence {
                      frame #0 {
                        n4192 = local write "34旅3"(TRUE) -> ()
                      }
                      frame #1 {
                        n4193 = property on="34旅3" class="Bool (strict)"("Visible"=TRUE) -> ()  [unwired: 2 in, 2 out]
                      }
                    }
                  }
                  frame 8 {
                    n4194 = flat-sequence {
                      frame #0 {
                        n4195 = local write "34旅4"(TRUE) -> ()
                      }
                      frame #1 {
                        n4196 = property on="34旅4" class="Bool (strict)"("Visible"=TRUE) -> ()  [unwired: 2 in, 2 out]
                      }
                    }
                  }
                }
                n4197 = case shown="1, Default" w3464 {
                  tunnel: w3465 -> [w3478 w3479 w3480 w3481]
                  frame 1, Default {
                    n4198 = local write "玩家一財產"(w3478) -> ()
                  }
                  frame 2 {
                    n4199 = local write "玩家二財產"(w3479) -> ()
                  }
                  frame 3 {
                    n4200 = local write "玩家三財產"(w3480) -> ()
                  }
                  frame 4 {
                    n4201 = local write "玩家四財產"(w3481) -> ()
                  }
                }
              }
              frame True {
                # "無主地"
                n4202 = call "購買土地.vi"() -> ("確定 2"=w3512:bool)  [unwired: 3 in]
                n4203 = case shown="True" w3512 {
                  tunnel: w3511 -> [_ w3516]
                  frame False {
                    # "不買"
                  }
                  frame True {
                    # "要買"
                    n4204 = local read "換誰?"() -> (w3517:dbl)
                    n4205 = case shown="4" w3517 {
                      tunnel: [w3544 w3545 w3546 w3547] -> w3515
